vi "Compare_CRC.vi"(0 "session in":refnum<k35>, 7 "Frame":string, 11 "error in (no error)":errorcluster) -> (4 "session out":refnum<k35>, 10 "CrcIsOk?":bool, 15 "error out":errorcluster)   [LabVIEW 2021]
panel:
  out "return value":string
  out "substring 2":string
  out "substring":string
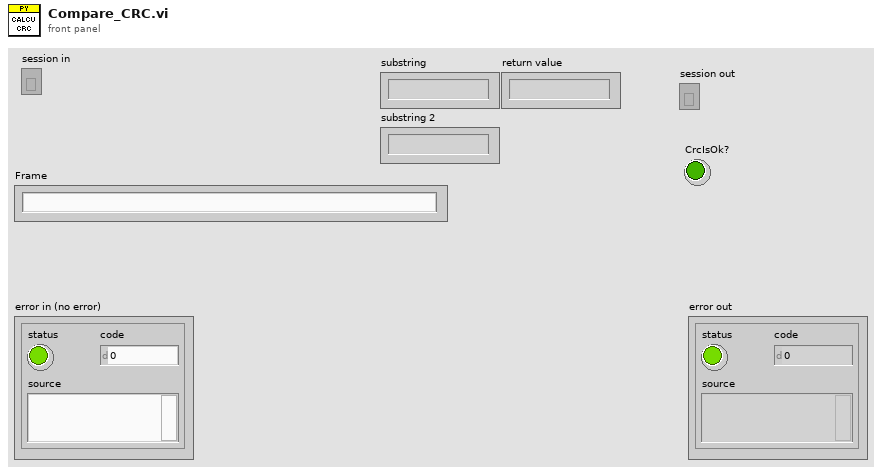
[diagram p1: front panel]
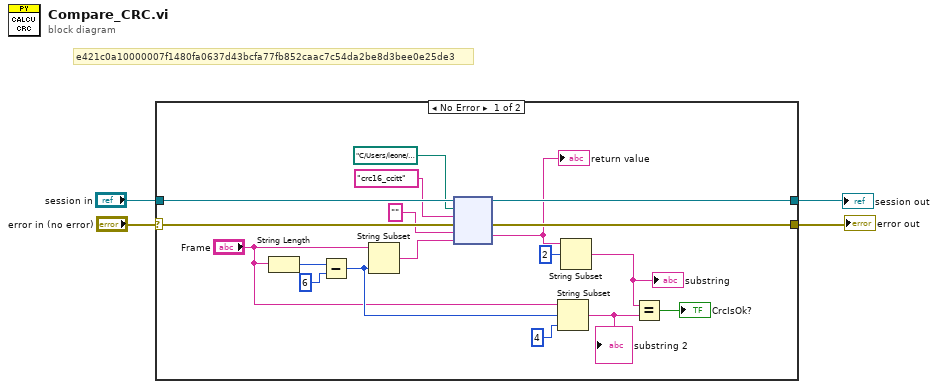
[diagram p0: block diagram]
diagram:
  # "e421c0a10000007f1480fa0637d43bcfa77fb852caac7c54da2be8d3bee0e25de3"
  n1 = case shown="No Error" "error in (no error)" {
    selector: "error in (no error)" -> [w18 w23]
    tunnel: "session in" -> [w22 w24]
    tunnel: [w21 w24] -> w4
    tunnel: [w20 w23] -> w3
    frame No Error {
      n2 = String Length(string="Frame") -> (length=w8:i32)
      n3 = Subtract(x=w8, y=6) -> (x-y=w6:i32)
      n4 = String Subset(string="Frame", length (rest)=w6) -> (substring=w7:string)  [unwired: 1 in]
      n5 = node(w22, path "C:/Users/leone/Desktop/GEA3/Serial-GEA/Crc.py" ("module path"), "crc16_ccitt" ("function name"), w18, "", w7) -> (w21:refnum<k35>, w20:errorcluster, w12:string)  [unwired: 1 in, 2 out]
      "return value" <- w12
      n6 = String Subset(string="Frame", offset (0)=w6, length (rest)=4 ("length (rest)")) -> (substring=w14:string)
      "substring 2" <- w14
      n7 = String Subset(string=w12, offset (0)=2) -> (substring=w10:string)  [unwired: 1 in]
      "substring" <- w10
      n8 = Equal?(x=w10, y=w14) -> (x = y?=→"CrcIsOk?":bool)
    }
    frame Error {
    }
  }
  "error out" <- w3
  "session out" <- w4
